vi "FP PC base station demo.vi"() -> ()   [LabVIEW 2014]
panel:
  out "circle\nradius":dbl=150.0
  out "Boat circle\ncenter":dbl[](array[numeric])
  in  "Data sent":string
  in  "stop":bool
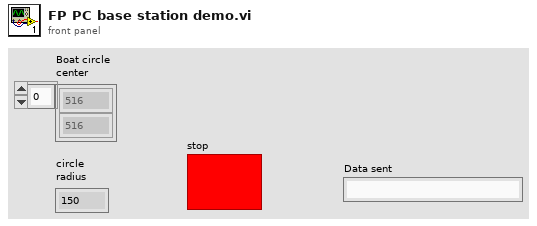
[diagram p1: front panel]
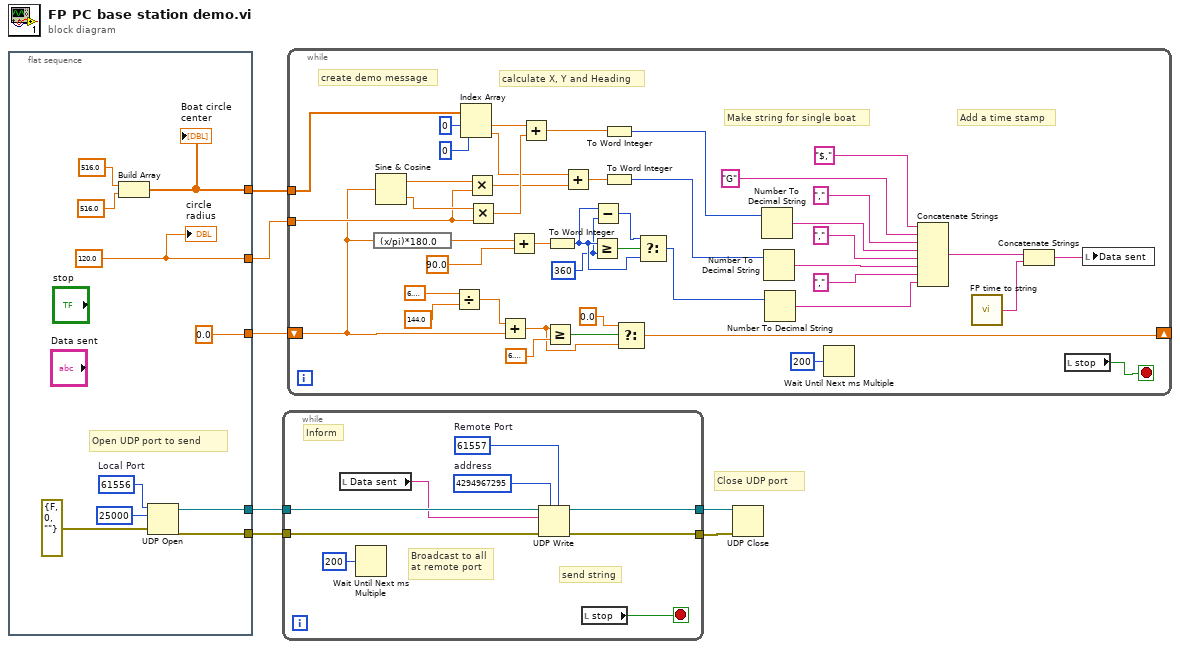
[diagram p0: block diagram]
diagram:
  # "Close UDP port"
  n1 = flat-sequence {
    tunnel: [w15] -> w5
    tunnel: [w14] -> w4
    tunnel: [w10] -> w3
    tunnel: [w9] -> w2
    tunnel: [0.0] -> w1
    frame #0 {
      w9 = 120.0
      w17 = u16 61556  # Local Port
      # "Open UDP port to send"
      n2 = Build Array(516.0, 516.0) -> (w10:dbl[])
      "Boat circle\ncenter" <- w10
      n3 = UDP Open(8:errorcluster {"status"=FALSE, "code"=0, "source"=""} ("error in (no error)"), 9:25000 ("timeout ms (25000)"), 11:w17) -> (port=w15:refnum<k16>, 0:w14:errorcluster)  [unwired: 3 out]
      "circle\nradius" <- w9
    }
  }
  n4 = while {
    tunnel: w5 -> [w26]
    tunnel: w4 -> [w25]
    tunnel: [w18] -> w7
    tunnel: [w19] -> w6
    stop <- w22 stop-if-true
    w24 = u16 61557  # Remote Port
    w21 = u32 4294967295  # address
    # "Inform"
    # "send string"
    # "Broadcast to all\nat remote port"
    n5 = local read "Data sent"() -> (w20:string)
    n6 = Wait Until Next ms Multiple(millisecond multiple=u32 200) -> ()  [unwired: 1 out]
    n7 = UDP Write(address=w21, port or service name=w24, connection ID=w26, data in=w20, 8:w25) -> (error out=w18:errorcluster, 3:w19:refnum<k16>)  [unwired: 1 out]
    n8 = local read "stop"() -> (w22:bool)
  }
  n9 = while {
    tunnel: w3 -> [w49]
    tunnel: w2 -> [w40]
    shift-right: [w50] -> _
    shift-left: w1 -> [w35]
    stop <- w62 stop-if-true
    w28 = i16 360 ("y")
    # "calculate X, Y and Heading"
    # "Add a time stamp"
    # "Make string for single boat"
    # "create demo message"
    n10 = expression code="(x/pi)*180.0" ("radians to degrees")(w35) -> (w34:dbl)
    n11 = Sine & Cosine(0:w35) -> (1:w41:dbl, 2:w46:dbl)
    n12 = Divide(x=6.283185307179586, y=144.0) -> (x/y=w55:dbl)
    n13 = Index Array(array=w49, index #1=0 ("index"), index #2=0) -> (element #1=w47:dbl, element #2=w38:dbl)
    n14 = Multiply(x=w41, y=w40) -> (x*y=w39:dbl)
    n15 = Multiply(x=w46, y=w40) -> (x*y=w45:dbl)
    n16 = Add(x=w55, y=w35) -> (x+y=w51:dbl)
    n17 = Add(x=w34, y=90.0) -> (x+y=w32:dbl)
    n18 = Add(x=w47, y=w45) -> (x+y=w44:dbl)
    n19 = Greater Or Equal?(x=w51, y=6.283185307179586) -> (x >= y?=w53:bool)
    n20 = To Word Integer(number=w32) -> (16bit integer=w29:i16)
    n21 = Add(x=w38, y=w39) -> (x+y=w37:dbl)
    n22 = Greater Or Equal?(x=w29, y=w28) -> (x >= y?=w31:bool)
    n23 = Subtract(x=w29, y=w28) -> (x-y=w27:i16)
    n24 = To Word Integer(number=w44) -> (16bit integer=w43:i16)
    n25 = To Word Integer(number=w37) -> (16bit integer=w36:i16)
    n26 = Select(t=0.0, s=w53, f=w51) -> (s? t:f=w50:dbl)
    n27 = Select(t=w27, s=w31, f=w29) -> (s? t:f=w30:i16)
    n28 = Number To Decimal String(number=w43) -> (decimal integer string=w70:string)  [unwired: 1 in]
    n29 = Number To Decimal String(number=w36) -> (decimal integer string=w68:string)  [unwired: 1 in]
    n30 = Number To Decimal String(number=w30) -> (decimal integer string=w66:string)  [unwired: 1 in]
    n31 = Wait Until Next ms Multiple(millisecond multiple=u32 200) -> ()  [unwired: 1 out]
    n32 = Concatenate Strings("$,", "G", ",", w70, ",", w68, ",", w66) -> (w61:string)
    n33 = call "FP time to string.vi"() -> ("time string"=w60:string)  [unwired: 1 in]
    n34 = Concatenate Strings(w61, w60) -> (w59:string)
    n35 = local read "stop"() -> (w62:bool)
    n36 = local write "Data sent"(w59) -> ()
  }
  n37 = UDP Close(connection ID=w6, 8:w7) -> ()  [unwired: 2 out]
